vi "read sysdef file.vi"(8 "error in (no error)":errorcluster, 9 "CD list in":variant, 10 "lookup in":variant, 11 "Path":path=path "C:/Users/Public/Documents/National Instruments/NI VeriStand 2014/Projects/Example/Sinewave Delay.nivssdf") -> (0 "error out":errorcluster, 1 "CD list out":variant, 2 "lookup out":variant)   [LabVIEW 2014]
uses:
  <vilib>/Utility/sysdir.llb/System Directory Type.ctl
  <vilib>/xml/Load XML File.vi
  <vilib>/xml/Close Reference(Node).vi
  <vilib>/xml/NI_XML.lvlib
  <resource>/objmgr/DOMUserDefRef.rc
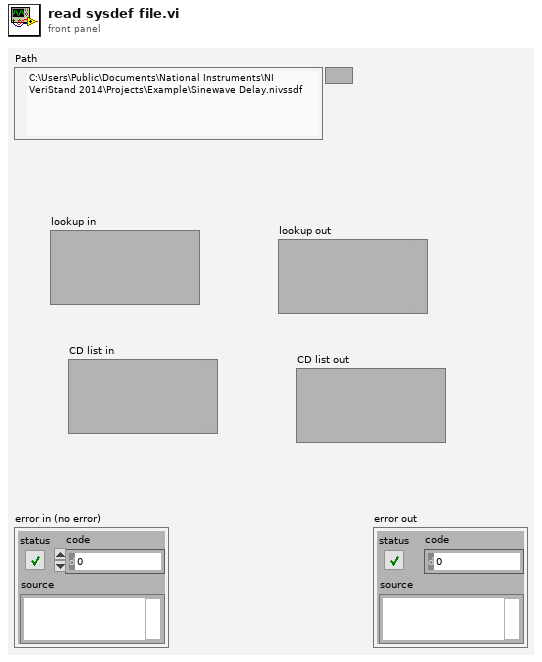
[diagram p1: front panel]
types:
  T1 = typedef "System Directory Type.ctl" = i32
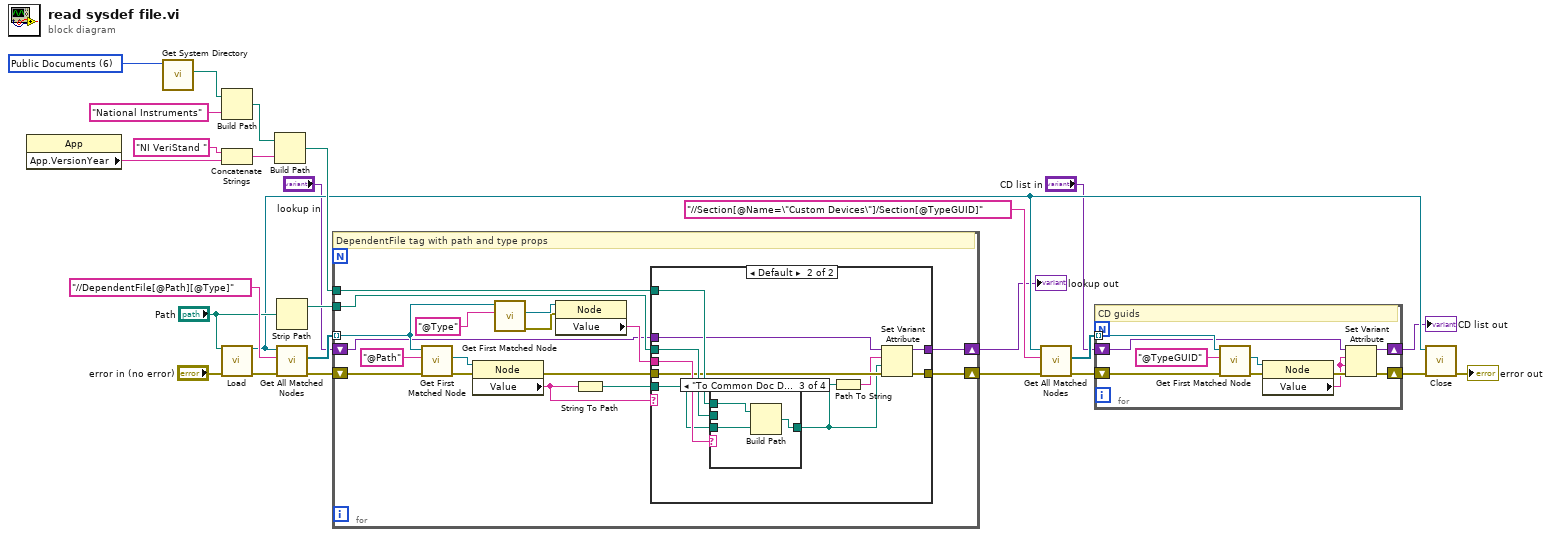
[diagram p0: block diagram]
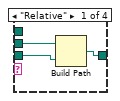
[diagram p3: hidden frame]
diagram:
  w18 = T1 6 items=["User Home"=0, "User Desktop"=1, "User Documents"=2, "User Application Data"=3, "User Preferences"=4, "User Temporary"=5, "Public Documents"=6, "Public Application Data"=7, "Public Preferences"=8, "Public Cache"=13, "System Core Libraries"=9, "System Installed Libraries"=10, "Application Files"=11, "Boot Volume Root"=12] ("system directory type")
  n1 = property class="App"() -> ("App.VersionYear"=w15:string)  [unwired: 2 in, 2 out]
  n2 = call <vilib>:"Get System Directory.vi"("system directory type"=w18) -> ("system directory"=w17:path)  [unwired: 10 in]
  n3 = Build Path(base path=w17, name or relative path="National Instruments") -> (appended path=w16:path)
  n4 = Concatenate Strings("NI VeriStand ", w15) -> (w12:string)
  n5 = call-poly <vilib>:"Load.vi"("path to XML document"="Path", "error in (no error)"="error in (no error)") -> ("DOM document out"=w9:refnum<k20>, "error out"=w24:errorcluster)  [unwired: 11 in, 1 out]
  n6 = Build Path(base path=w16, name or relative path=w12) -> (appended path=w11:path)
  n7 = Strip Path(path="Path") -> (stripped path=w19:path)  [unwired: 1 out]
  n8 = call <vilib>:"Get All Matched Nodes.vi"("error in (no error)"=w24, "XPath expression"="//DependentFile[@Path][@Type]", "node in"=w9) -> ("error out"=w21:errorcluster, "node result array"=w22:refnum<k20>[])  [unwired: 6 in, 1 out]
  n9 = for {
    tunnel: w22 -> [w35] mode=indexing
    shift-right: [w29] -> w10
    shift-left: w21 -> [w43]
    tunnel: w19 -> [w32]
    tunnel: w11 -> [w31]
    shift-right: [w27] -> w1
    shift-left: "lookup in" -> [w28]
    # "DependentFile tag with path and type props"
    n10 = call <vilib>:"Get First Matched Node.vi"("error in (no error)"=w43, "XPath expression"="@Path", "node in"=w35) -> ("error out"=w41:errorcluster, "node result"=w40:refnum<k20>)  [unwired: 6 in, 1 out]
    n11 = property class="Node"(reference=w40, error in=w41) -> (error out=w30:errorcluster, "Value"=w39:string)  [unwired: 1 out]
    n12 = call <vilib>:"Get First Matched Node.vi"("XPath expression"="@Type", "node in"=w35) -> ("error out"=w37:errorcluster, "node result"=w38:refnum<k20>)  [unwired: 7 in, 1 out]
    n13 = property class="Node"(reference=w38, error in=w37) -> ("Value"=w34:string)  [unwired: 2 out]
    n14 = String To Path(string=w39) -> (path=w33:path)
    n15 = case shown="Default" w39 {
      tunnel: w34 -> [_ w55]
      tunnel: w33 -> [_ w54]
      tunnel: w32 -> [_ w53]
      tunnel: w31 -> [_ w52]
      tunnel: w30 -> [w45 w50]
      tunnel: [w45 w51] -> w29
      tunnel: w28 -> [w44 w47]
      tunnel: [w44 w46] -> w27
      frame "\u0000" {
      }
      frame Default {
        n16 = case shown="\"To Common Doc Dir\"" w55 {
          tunnel: [w57 w59 w60 w63] -> w49
          tunnel: w54 -> [w56 w59 w61 w63]
          tunnel: w53 -> [w58 _ _ _]
          tunnel: w52 -> [_ _ w62 _]
          frame "Relative" {
            n17 = Build Path(base path=w58, name or relative path=w56) -> (appended path=w57:path)
          }
          frame "Absolute" {
          }
          frame "To Common Doc Dir" {
            n18 = Build Path(base path=w62, name or relative path=w61) -> (appended path=w60:path)
          }
          frame "", Default {
          }
        }
        n19 = Path To String(path=w49) -> (string=w48:string)
        n20 = Set Variant Attribute(Variant=w47, name=w48, value=w49, error in=w50) -> (Variant out=w46:variant, error out=w51:errorcluster)  [unwired: 1 out]
      }
    }
  }
  "lookup out" <- w1
  n21 = call <vilib>:"Get All Matched Nodes.vi"("error in (no error)"=w10, "XPath expression"="//Section[@Name=\"Custom Devices\"]/Section[@TypeGUID]", "node in"=w9) -> ("error out"=w6:errorcluster, "node result array"=w5:refnum<k20>[])  [unwired: 6 in, 1 out]
  n22 = for {
    shift-right: [w67] -> w7
    shift-left: w6 -> [w69]
    tunnel: w5 -> [w68] mode=indexing
    shift-right: [w65] -> w4
    shift-left: "CD list in" -> [w66]
    # "CD guids"
    n23 = call <vilib>:"Get First Matched Node.vi"("error in (no error)"=w69, "XPath expression"="@TypeGUID", "node in"=w68) -> ("error out"=w72:errorcluster, "node result"=w73:refnum<k20>)  [unwired: 6 in, 1 out]
    n24 = property class="Node"(reference=w73, error in=w72) -> (error out=w70:errorcluster, "Value"=w64:string)  [unwired: 1 out]
    n25 = Set Variant Attribute(Variant=w66, name=w64, value=w64, error in=w70) -> (Variant out=w65:variant, error out=w67:errorcluster)  [unwired: 1 out]
  }
  "CD list out" <- w4
  n26 = call-poly <vilib>:"Close.vi"("error in (no error)"=w7, "node"=w9) -> ("error out"=→"error out":errorcluster)  [unwired: 7 in]
